vi "9613 Empty Section Name--error.vi"(8 "error in":errorcluster) -> (0 "error out":errorcluster)   [LabVIEW 2019, in "Electronic Datasheet.lvlib"]
uses:
  Electronic Datasheet.lvlib
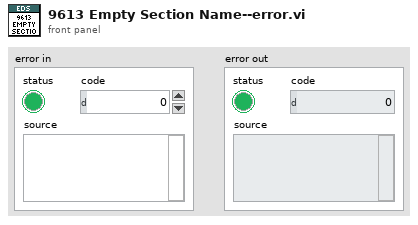
[diagram p1: front panel]
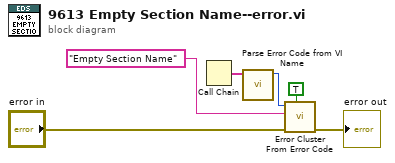
[diagram p0: block diagram]
diagram:
  n1 = Call Chain() -> (call chain=w3:string[])
  n2 = call "Parse Error Code from VI Name.vi"("Call Chain"=w3) -> ("Error Code"=w2:i32)  [unwired: 10 in]
  n3 = call <vilib>:"Error Cluster From Error Code.vi"("show call chain? (False)"=TRUE, "error in (no error)"="error in", "error message (\"\")"="Empty Section Name" ("error message (\"\")"), "error code (0)"=w2) -> ("error out"=→"error out":errorcluster)  [unwired: 5 in]
